vi "Inverse FFT.vi"   [LabVIEW 2020, in "NI_AALPro.lvlib"]
doc: "Computes the inverse discrete Fourier transform (IDFT) of the input sequence <B>FFT {X}</B>. You must manually select the polymorphic instance you want to use."
uses:
  <vilib>/Analysis/NI_AALPro.lvlib
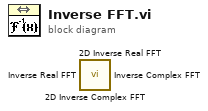
[diagram p0: block diagram]
diagram:
  n1 = call <vilib>:"2D Inverse Complex FFT.vi"() -> ()  [unwired: 10 in, 2 out]
  n2 = call <vilib>:"2D Inverse Real FFT.vi"() -> ()  [unwired: 10 in, 2 out]
  n3 = call <vilib>:"Inverse Real FFT.vi"() -> ()  [unwired: 10 in, 2 out]
  n4 = call <vilib>:"Inverse Complex FFT.vi"() -> ()  [unwired: 10 in, 2 out]
